vi "Continuous B sweep.vi"(7 "Rate (T/min)":dbl=0.028 min=0.0 max=0.2, 8 "error in (no error)":errorcluster, 9 "Simulate/Run":enum16{"simulate mode", "run mode"}(ring)=enum."run mode", 10 "Min (start)":dbl=7.0 min=-8.0 max=8.0, 11 "Max (end)":dbl=-7.0 min=-8.0 max=8.0) -> (0 "error out":errorcluster)   [LabVIEW 2016, in "SweepControl.lvclass"]
uses:
  SweepControl.lvclass
  Typedefs/Enum - Experiments.ctl
  Typedefs/Continuous B Sweep JSON--Cluster.ctl
  <userlib>/LevyLab/Levylab Instruments/Instrument Types/Cryostat/Instrument.Cryostat.lvclass
  Transport/Transport.lvclass
  Control Experiment/Control Experiment SM.lvclass
  <userlib>/LevyLab/Krohn Hite 7008/Instrument.KH7008.lvclass
  <userlib>/LevyLab/Lockin-Multichannel/Instrument.Lockin/Instrument.Lockin.lvclass
  Control Experiment/Typedefs/Instruments--cluster.ctl
  <userlib>/LevyLab/Krohn Hite 7008/typedefs/Input Configuration-Enum.ctl
  <userlib>/LevyLab/Krohn Hite 7008/typedefs/Shunt-Enum.ctl
  <userlib>/LevyLab/Krohn Hite 7008/typedefs/Gain-Enum.ctl
  <userlib>/LevyLab/Krohn Hite 7008/typedefs/Channel-Enum.ctl
  Control Experiment/Typedefs/Wiring Description--cluster.ctl
  Control Experiment/Typedefs/Instrument--enum.ctl
  Control Experiment/Typedefs/Experiment Description--cluster.ctl
  <userlib>/LevyLab/Levylab Instruments/Instrument Types/VSource/Instrument.VSource.lvclass
  <userlib>/LevyLab/Levylab Instruments/Instrument Types/VNA/Instrument.VNA.lvclass
  <userlib>/LevyLab/Levylab Instruments/Instrument Types/Strain/Instrument.Strain.lvclass
  <userlib>/LevyLab/Levylab Instruments/Instrument Types/Optical Delay Line/Instrument.OpticalDelayLine.lvclass
  <userlib>/LevyLab/Levylab Instruments/Instrument Types/CBridge/Instrument.CBridge.lvclass
  <userlib>/LevyLab/Krohn Hite 7008/typedefs/Coupling-Enum.ctl
  <userlib>/LevyLab/Krohn Hite 7008/typedefs/Filter-Enum.ctl
  <userlib>/LevyLab/Krohn Hite 7008/typedefs/SetAll-Cluster.ctl
  <userlib>/LevyLab/Krohn Hite 7008/typedefs/SetAll-Array.ctl
  <userlib>/LevyLab/Lockin-Multichannel/Lockin.DAQ/Typedefs/REF-cluster.ctl
  <userlib>/LevyLab/Lockin-Multichannel/Lockin.DAQ/Lockin.DAQ.lvclass
  <userlib>/LevyLab/Lockin-Multichannel/Lockin.DAQ/Typedefs/Function-enum.ctl
  <userlib>/LevyLab/Lockin-Multichannel/Lockin.DAQ/Typedefs/AO-cluster.ctl
  Typedefs/Lockin Sweep--Cluster.ctl
panel:
  in  "Sweep Lockin Array":T1[](array[typedef]) {"Sweep End (V)" format="%#_6p"; "Sweep Start (V)" format="%#_6p"}
  out "Current Setpoint":dbl
  in  "Experiment Folder":string="4L4Lockinfieldsweep"
  in  "Experiment subVI":T2
  in  "Experiment Description":string="SA03036H\nsweep Vsg:-150m to 700m, 500u steps\nB 7T to -7T\nVbg =-3.9V\nT: 50mK\n\nlockin\n\nI+/-: 4/28 200uV ac+ 250u dc bias, 13Hz\nV1+/-: 3/27\nV2+/- 2/6\nV3+/V3-: 7/8\nVsg: 1\nVbg :26\n\ntc 300ms order 2"
  in  "OK":bool
  out "time (minutes)":dbl
  out "ETA":timestamp=timestamp(3224621726.1089997 s since 1904-01-01) caption="Timestamp" format="%<%m/%d/%Y %I:%M:%S %p>T"
  out "time (hours)":dbl
  out "Current Step":i32
  in  "Function":enum16{"Ramp", "Triangle", "Sine"}(ring)
  in  "Phase":dbl
  in  "Cycles (1,2,...)":i32=1 min=1 step=1
  in  "step size":dbl=14.0 format="%.4f"
  out "B Field Graph":cluster{i32[], dbl[]}[](graph)
  in  "stop":bool
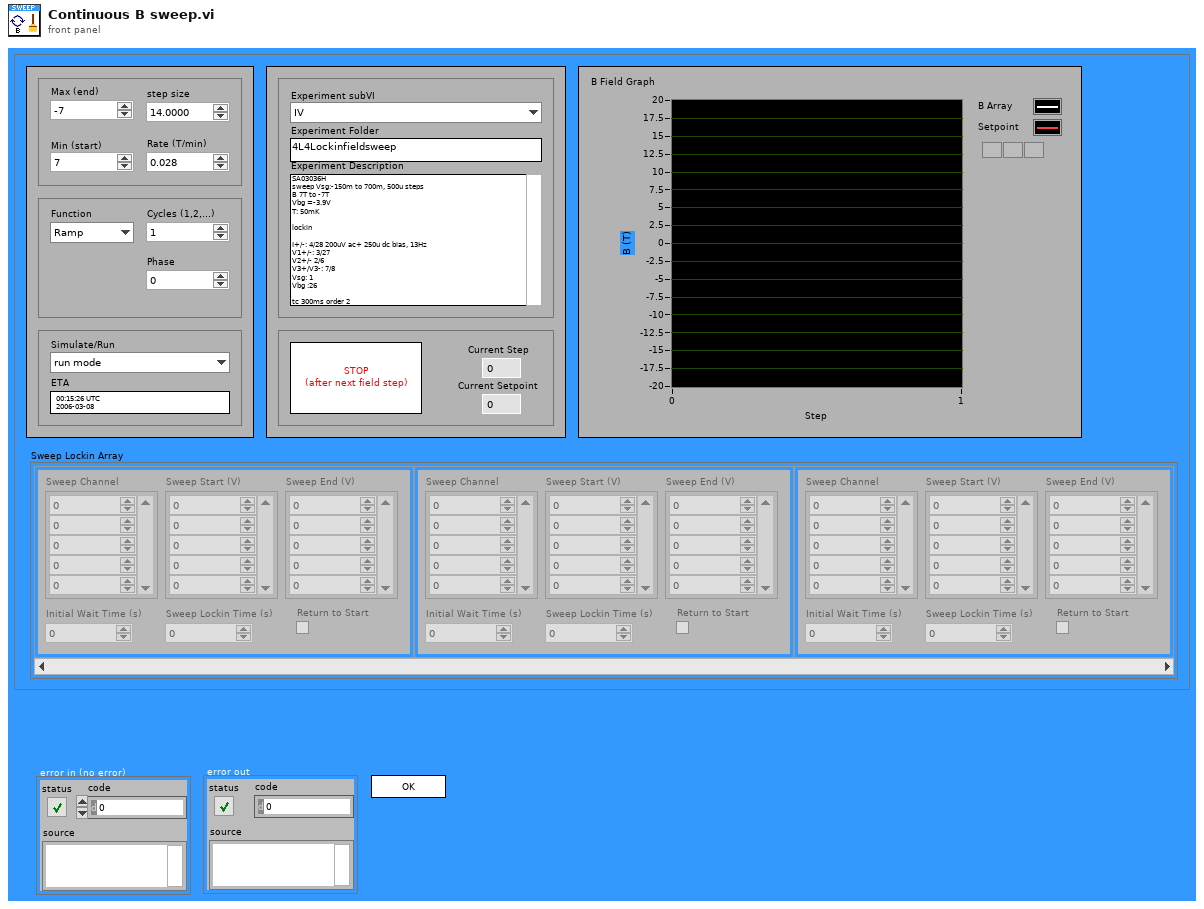
[diagram p1: front panel]
types:
  T1 = typedef "SweepControl.lvclass/Lockin Sweep--Cluster.ctl" = cluster{"Sweep Lockin Time (s)":dbl, "Initial Wait Time (s)":dbl, "Sweep Channel":i32[], "Sweep Start (V)":dbl[], "Sweep End (V)":dbl[], "Return to Start":bool}
  T2 = typedef "SweepControl.lvclass/Enum - Experiments.ctl" = enum16{"IV", "IV_Fast", "IV_Sweep", "THz_DelayLine", "Lockin_Vsg", "Lockin_Sweep", "Lockin_Time", "AI WFM time", "Lockin (experimental)"}
  T3 = enum32{"Invalid", "Standard", "Closed", "Hidden", "Minimized", "Maximized"}
  T4 = enum32{"invalid app kind", "Development System", "Run Time System", "Student Edition", "Embedded LabVIEW", "Evaluation", "Custom"}
  T5 = typedef "Control Experiment SM.lvclass/Instruments--cluster.ctl" = cluster{"KH7008":refnum<class "Instrument.KH7008.lvclass">[], "Lockin":refnum<class "Instrument.Lockin.lvclass">, "Temperature":refnum<class "Instrument.Cryostat.lvclass">, "Magnet":refnum<class "Instrument.Cryostat.lvclass">, "Rotator":refnum<class "Instrument.Cryostat.lvclass">, "Level":refnum<class "Instrument.Cryostat.lvclass">, "Capacitance Bridge":refnum<class "Instrument.CBridge.lvclass">, "Optical Delay Line":refnum<class "Instrument.OpticalDelayLine.lvclass">, "Strain Cell":refnum<class "Instrument.Strain.lvclass">, "VNA":refnum<class "Instrument.VNA.lvclass">, "Voltage Source":refnum<class "Instrument.VSource.lvclass">}
  T6 = cluster{"Core":cluster{"Current VI Reference":refnum<vi>, "Close Panel on Exit?":bool}, "SweepControl":refnum<class "SweepControl.lvclass">, "B field values":dbl[], "Sweep rate (T/min)":dbl, "Transport":refnum<class "Transport.lvclass">, "Instruments":T5, "Notifier":refnum<notifier>}
  T7 = cluster{"Current VI Reference":refnum<vi>, "Close Panel on Exit?":bool}
  T8 = typedef "SweepControl.lvclass/Continuous B Sweep JSON--Cluster.ctl" = cluster{"Continuous B Sweep":cluster{"Experiment":T2, "B field values":dbl[]}, "Experiment Description":T9, "Wiring Configuration":T11, "Lockin":cluster{"Channels: AO":T12, "Channels: Lockin":T14}, "Krohn Hite":cluster{"Channel Setting":T15}}
  T9 = typedef "Control Experiment SM.lvclass/Experiment Description--cluster.ctl" = cluster{"User":string, "Device":string, "Device Path":path, "Device Description":string, "Experiment Path":path, "Experiment Description":string, "Instrument":T10, "Sweep":cluster{"key":string, "value":variant}[], "Device Description JSON":string, "Experiment Description JSON":string}
  T10 = typedef "Control Experiment SM.lvclass/Instrument--enum.ctl" = enum16{"----- AFM/EBL -----", "AGILENT", "CYPHER", "Gemini2", "JEOL", "MFP3D", "----- Cryostat -----", "CF900", "DR200", "MNK", "PPMS 1", "PPMS 2", "PPMS 3", "----- Optics -----", "THz 1", "THz 2"}
  T11 = typedef "Control Experiment SM.lvclass/Wiring Description--cluster.ctl" = cluster{"Lockin Ch":i32[], "KH":cluster{"Electrodes":string[], "Labels":string[]}, "not KH":cluster{"Electrodes":string[], "Labels":string[]}}
  T12 = typedef "Lockin.DAQ.lvclass/AO-cluster.ctl" = cluster{"Ch":i32[], "Amp (V)":dbl[], "DC (V)":dbl[], "f (Hz)":dbl[], "Phase (°)":dbl[], "Function":T13[], "Sweep?":bool[]}
  T13 = typedef "Lockin.DAQ.lvclass/Function-enum.ctl" = enum16{"Sine", "Triangle", "Square", "Sawtooth"}
  T14 = typedef "Lockin.DAQ.lvclass/REF-cluster.ctl" = cluster{"Ch":i32[], " f (Hz)":dbl[], "Phase (°)":dbl[], "TC (s)":dbl[], "order":i32[]}
  T15 = typedef "Instrument.KH7008.lvclass/SetAll-Array.ctl" = T16[]
  T16 = typedef "Instrument.KH7008.lvclass/SetAll-Cluster.ctl" = cluster{"Channel":T17, "Gain":T18, "Bandwidth Filter":T19, "Shunt Resistor":T20, "Coupling":T21, "Input Config":T22}
  T17 = typedef "Instrument.KH7008.lvclass/Channel-Enum.ctl" = enum16{"Channel 1", "Channel 2", "Channel 3", "Channel 4", "Channel 5", "Channel 6", "Channel 7", "Channel 8"}
  T18 = typedef "Instrument.KH7008.lvclass/Gain-Enum.ctl" = enum16{"1x", "10x", "100x", "1000x"}
  T19 = typedef "Instrument.KH7008.lvclass/Filter-Enum.ctl" = enum16{"OFF", "ON"}
  T20 = typedef "Instrument.KH7008.lvclass/Shunt-Enum.ctl" = enum16{"Open", "50 Ohms", "500 Ohms", "5k Ohms", "50k Ohms", "10M Ohm"}
  T21 = typedef "Instrument.KH7008.lvclass/Coupling-Enum.ctl" = enum16{"AC", "DC"}
  T22 = typedef "Instrument.KH7008.lvclass/Input Configuration-Enum.ctl" = enum16{"Ground", "SE+ (-gnd)", "SE- (+gnd)", "Differential"}
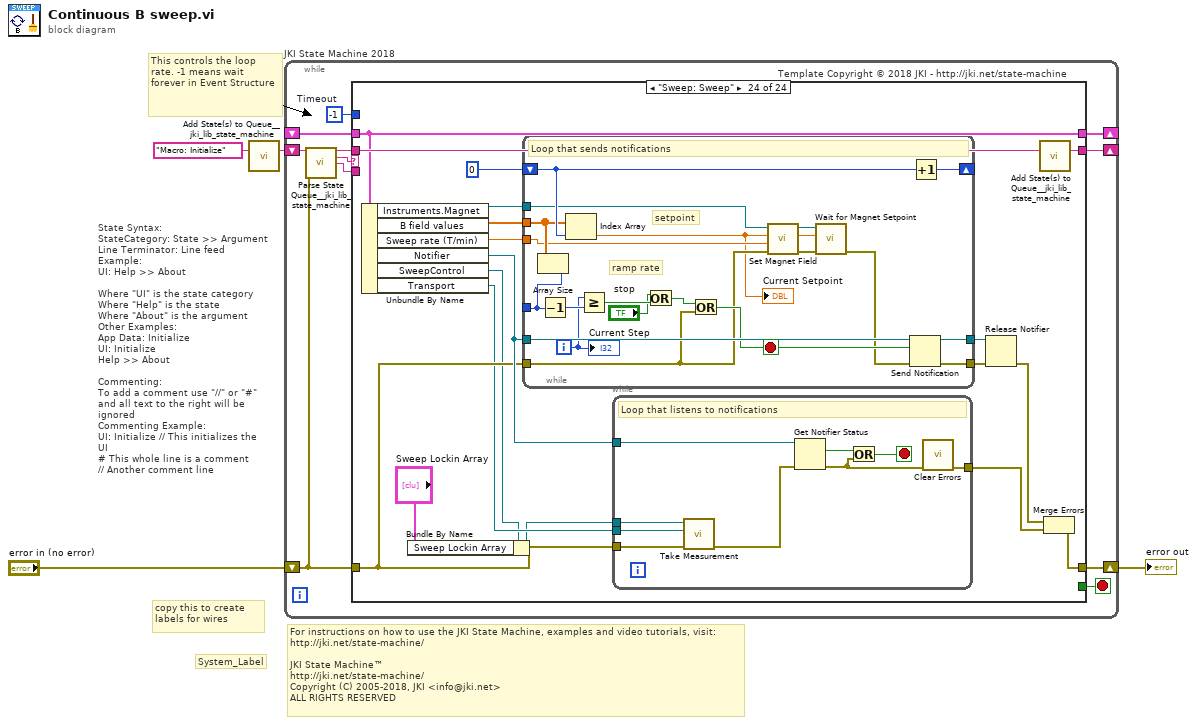
[diagram p0: block diagram]
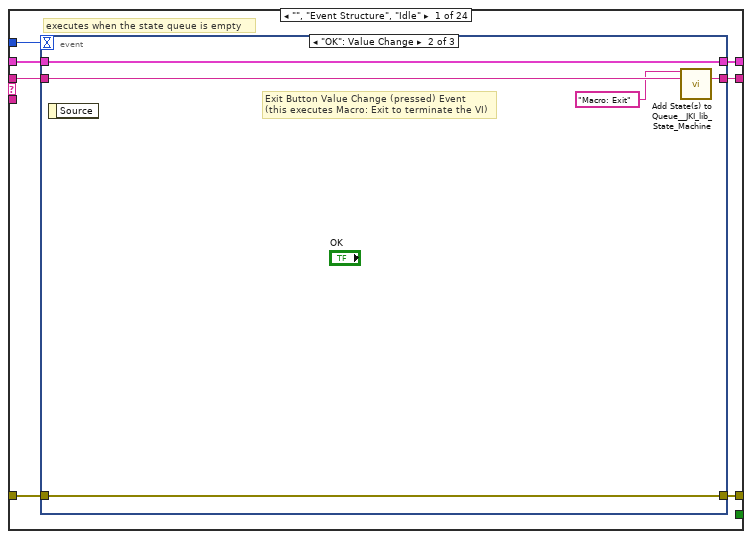
[diagram p2: hidden frame]
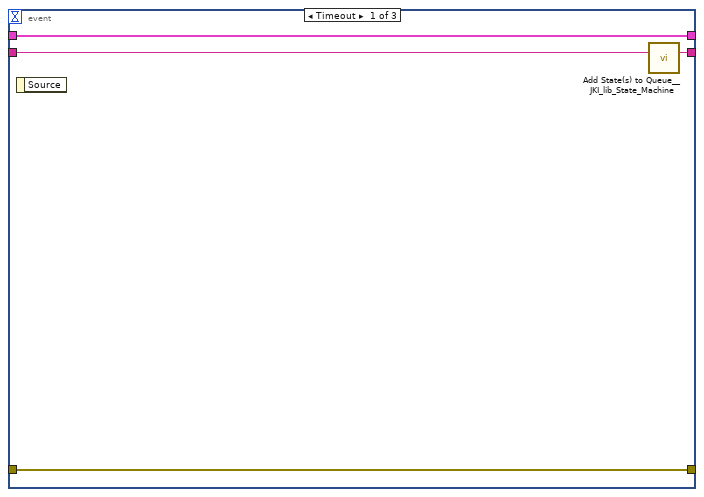
[diagram p3: hidden frame]
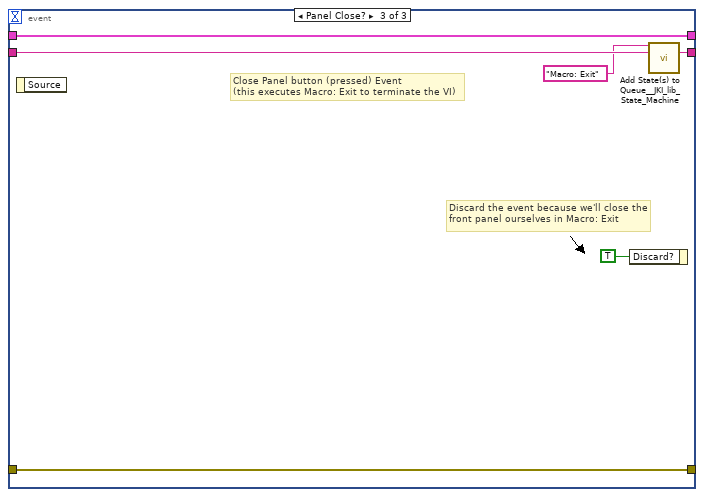
[diagram p4: hidden frame]
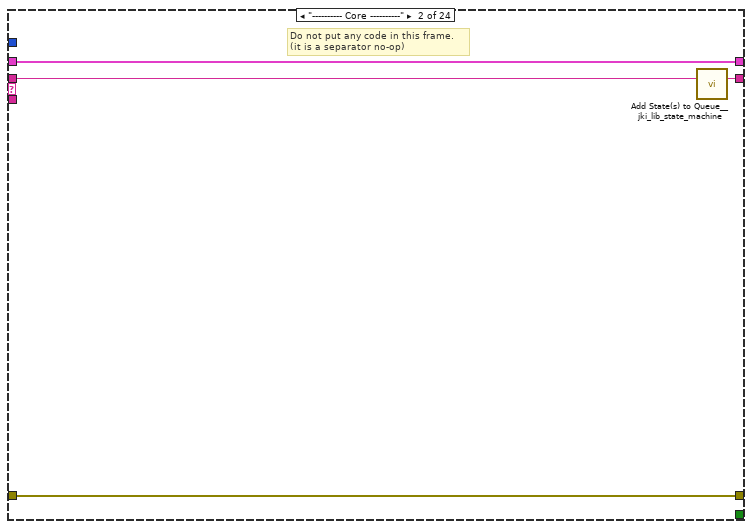
[diagram p5: hidden frame]
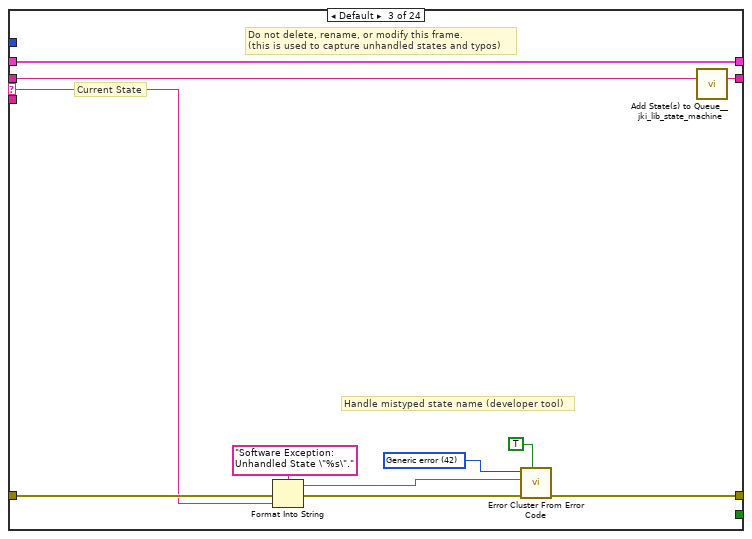
[diagram p6: hidden frame]
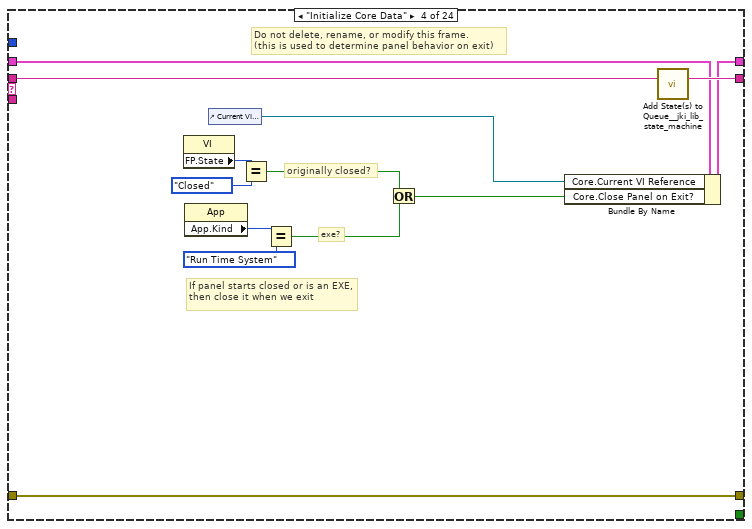
[diagram p7: hidden frame]
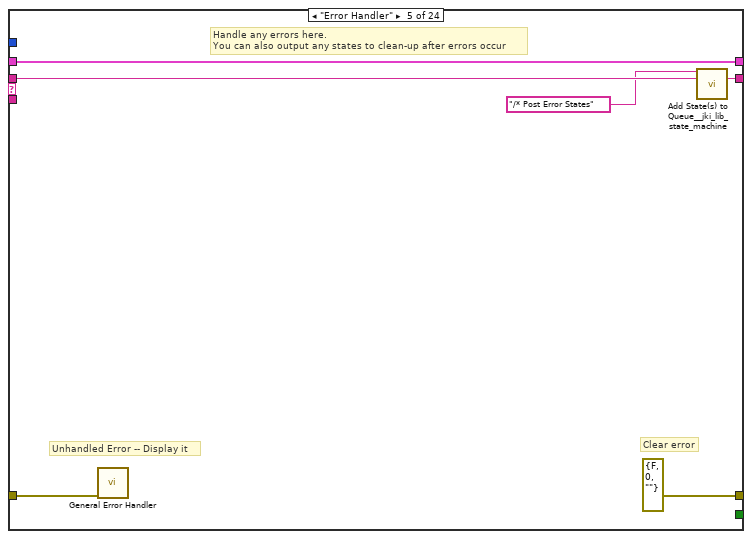
[diagram p8: hidden frame]
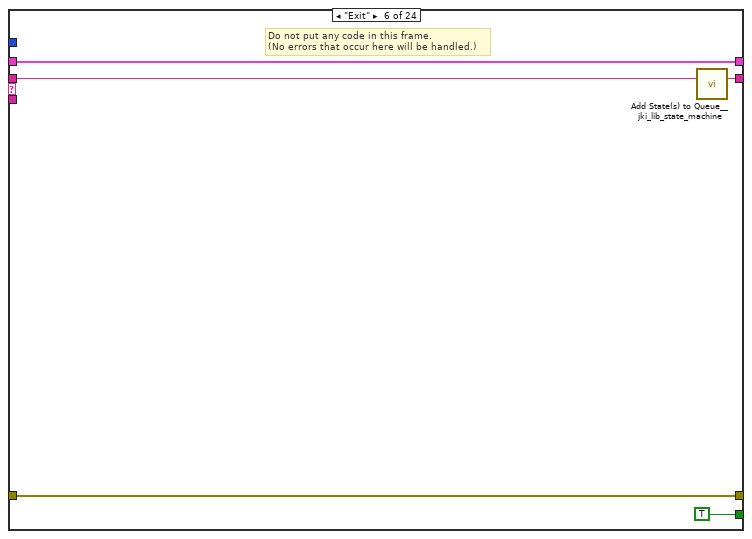
[diagram p9: hidden frame]
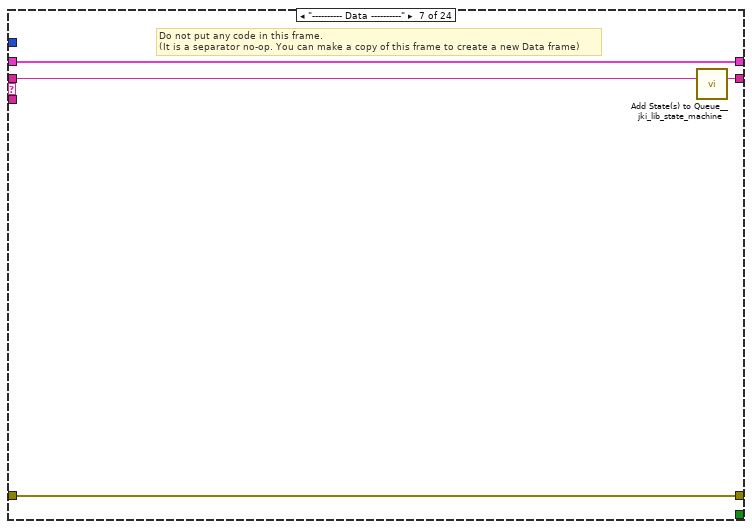
[diagram p10: hidden frame]
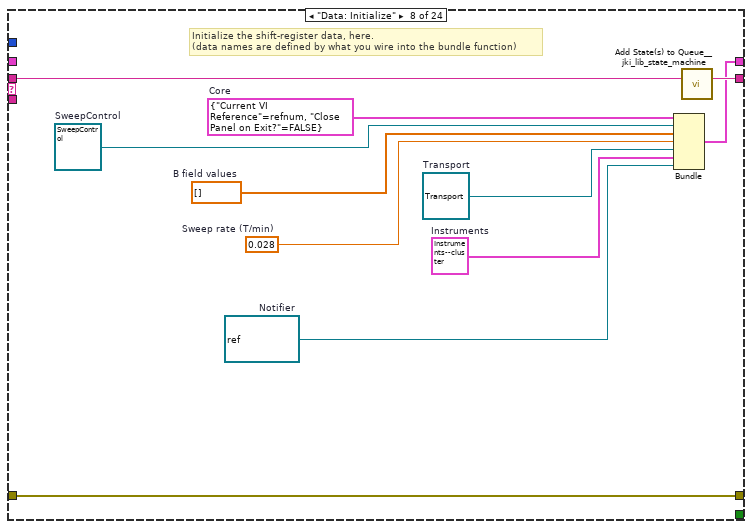
[diagram p11: hidden frame]
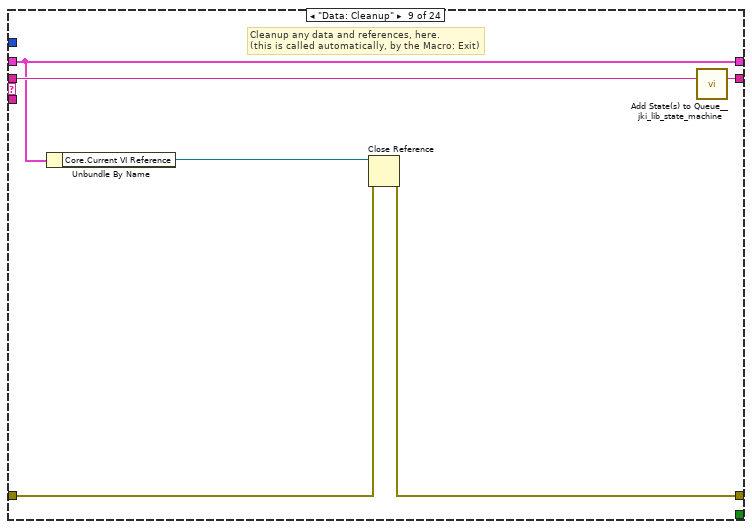
[diagram p12: hidden frame]
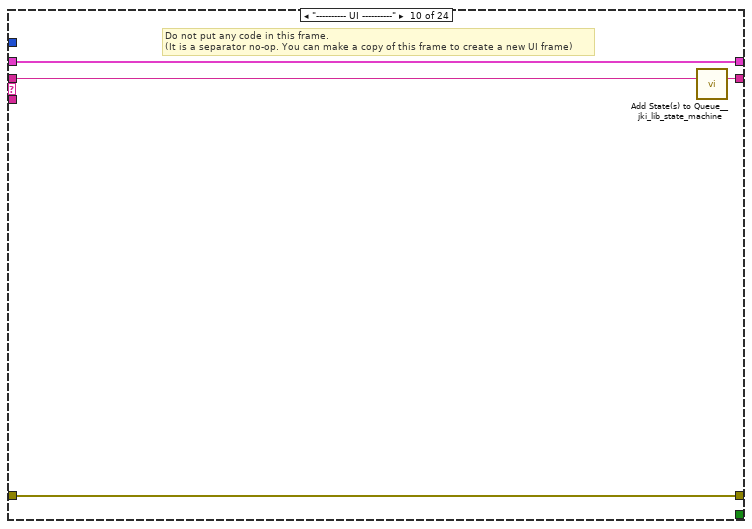
[diagram p13: hidden frame]
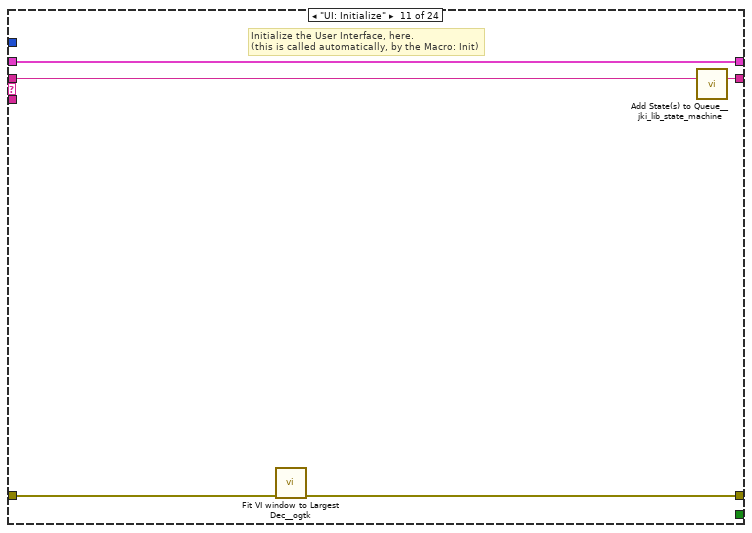
[diagram p14: hidden frame]
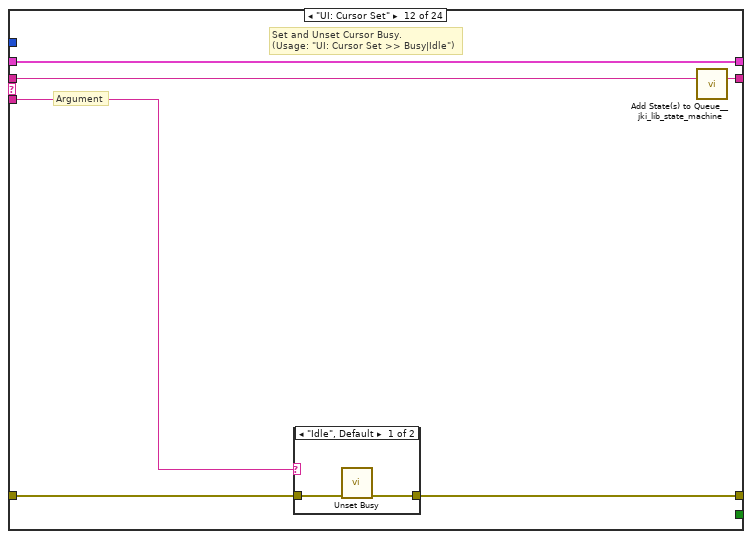
[diagram p15: hidden frame]
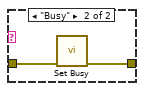
[diagram p16: hidden frame]
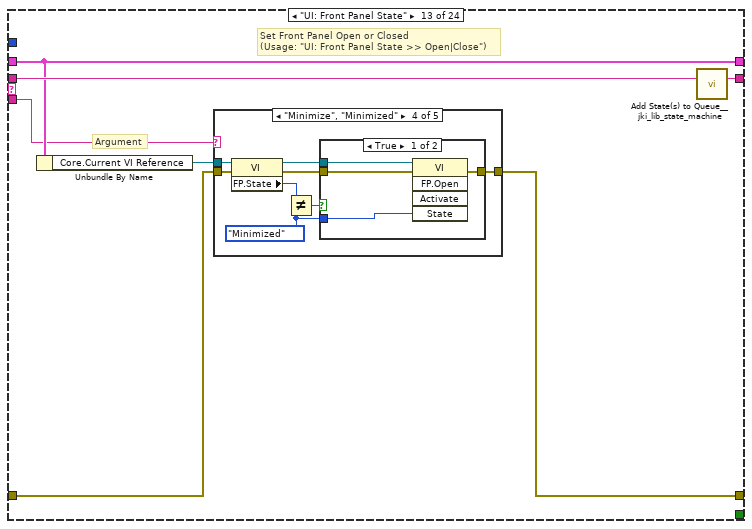
[diagram p17: hidden frame]
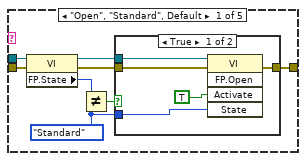
[diagram p18: hidden frame]
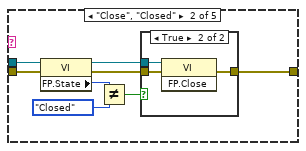
[diagram p20: hidden frame]
diagram:
  # "For instructions on how to use the JKI State Machine, examples and video tutorials, visit:\nhttp://jki.net/state-machine/\n\nJKI State Machine™\nhttp://jki.net/state-machine/\nCopyright (C) 2005-2018, JKI <info@jki.net>\nALL RIGHTS RESERVED"
  # "State Syntax:\nStateCategory: State >> Argument\nLine Terminator: Line feed\nExample:\nUI: Help >> About\n\nWhere \"UI\" is the state category\nWhere \"Help\" is the state\nWhere \"About\" is the argument\nOther Examples:\nApp Data: Initialize\nUI: Initialize\nHelp >> About\n\nCommenting:\nTo add a comment use \"//\" or \"#\" and all text to the right will be ignored\nCommenting Example:\nUI: Initialize // This initializes the UI\n# This whole line is a comment\n// Another comment line"
  # "copy this to create labels for wires"
  # "This controls the loop rate. -1 means wait forever in Event Structure"
  # "System_Label"
  n1 = call <vilib>:"Add State(s) to Queue__jki_lib_state_machine.vi"("State(s) in (\"\")"="Macro: Initialize") -> ("States Out"=w4:string)  [unwired: 14 in]
  n2 = while "JKI State Machine 2018" {
    shift-right: [w8] -> _
    shift-left: _ -> [w7]
    shift-right: [w11] -> w1
    shift-left: "error in (no error)" -> [w5]
    shift-right: [w10] -> _
    shift-left: w4 -> [w12]
    stop <- w9 stop-if-true
    w6 = -1  # Timeout
    # "Template Copyright © 2018 JKI - http://jki.net/state-machine"
    n3 = call <vilib>:"Parse State Queue__jki_lib_state_machine.vi"("State Queue"=w12, "Error In (no error)"=w5) -> ("Remaining States"=w14:string, "Current State"=w15:string, "Arguments"=w13:string)  [unwired: 11 in]
    n4 = case shown="\"Sweep: Sweep\"" w15 {
      selector: w15 -> [_ _ w42 _ _ _ _ _ _ _ _ _ _ _ _ _ _ _ _ _ _ _ _ _]
      tunnel: w14 -> [w22 w41 w46 w65 w71 w76 w80 w91 w97 w101 w106 w112 w123 w192 w197 w203 w215 w219 w238 w260 w274 w300 w321 w357]
      tunnel: w13 -> [_ _ _ _ _ _ _ _ _ _ _ w107 w117 _ _ _ _ _ _ _ _ _ _ _]
      tunnel: w7 -> [w20 w38 w44 w58 w68 w74 w77 _ w92 w98 w104 w110 w119 w189 w194 w200 w212 w216 w228 w244 w269 w298 w308 w349]
      tunnel: [w19 w39 w48 w62 errorcluster {"status"=FALSE, "code"=0, "source"=""} ("error out") w73 w78 w88 w93 w99 w102 w108 w120 w190 w195 w201 w213 w217 w226 w248 w267 w295 w319 w350] -> w11
      tunnel: w5 -> [w18 w39 w47 w62 w67 w73 w78 w88 w94 w99 w103 w109 w121 w190 w195 w201 w213 w217 w226 w249 w268 w282 w319 w344]
      tunnel: [w21 w40 w45 w64 w70 w75 w79 w90 w96 w100 w105 w111 w122 w191 w196 w202 w214 w218 w237 w259 w273 w299 w320 w356] -> w10
      tunnel: [_ _ _ _ _ TRUE _ _ _ _ _ _ _ _ _ _ _ _ _ _ _ _ _ _] -> w9
      tunnel: [w17 w38 w44 w63 w68 w74 w77 w89 w92 w98 w104 w110 w119 w189 w194 w200 w212 w216 w236 w243 w270 w298 w308 w349] -> w8
      tunnel: w6 -> [w16 _ _ _ _ _ _ _ _ _ _ _ _ _ _ _ _ _ _ _ _ _ _ _]
      frame "", "Event Structure", "Idle" {
        # "executes when the state queue is empty"
        n5 = event shown="[1] \"OK\": Value Change" {
          selector: _ -> [_ _ _]
          dyn-events: _ -> [_ _ _]
          timeout: w16 -> [_ _ _]
          tunnel: w22 -> [w26 w31 w37]
          tunnel: [w25 w30 w36] -> w21
          tunnel: w20 -> [w23 w28 w34]
          tunnel: [w24 w29 w35] -> w19
          tunnel: w18 -> [w24 w29 w35]
          tunnel: [w23 w28 w34] -> w17
          event Timeout {
            n6 = event-data() -> ()  [unwired: 1 in, 1 out]
            n7 = call <vilib>:"Add State(s) to Queue__JKI_lib_State_Machine.vi"("State(s) in (\"\")"=w26) -> ("States Out"=w25:string)  [unwired: 14 in]
          }
          event "OK": Value Change {
            # "Exit Button Value Change (pressed) Event\n(this executes Macro: Exit to terminate the VI)"
            n8 = event-data() -> ()  [unwired: 1 in, 1 out]
            n9 = call <vilib>:"Add State(s) to Queue__JKI_lib_State_Machine.vi"("State(s) in Front (\"\")"="Macro: Exit", "State(s) in (\"\")"=w31) -> ("States Out"=w30:string)  [unwired: 13 in]
          }
          event Panel Close? {
            # "Discard the event because we'll close the front panel ourselves in Macro: Exit"
            # "Close Panel button (pressed) Event\n(this executes Macro: Exit to terminate the VI)"
            n10 = event-data() -> ()  [unwired: 1 in, 1 out]
            n11 = event-data("Discard?"=TRUE) -> ()  [unwired: 1 in, 1 out]
            n12 = call <vilib>:"Add State(s) to Queue__JKI_lib_State_Machine.vi"("State(s) in Front (\"\")"="Macro: Exit", "State(s) in (\"\")"=w37) -> ("States Out"=w36:string)  [unwired: 13 in]
          }
        }
      }
      frame "---------- Core ----------" {
        # "Do not put any code in this frame.\n(it is a separator no-op)"
        n13 = call <vilib>:"Add State(s) to Queue__jki_lib_state_machine.vi"("State(s) in (\"\")"=w41) -> ("States Out"=w40:string)  [unwired: 14 in]
      }
      frame Default {
        w51 = 42 items=["No error", "Argument error", "Memory is full", "Out of zone", "End of file", "File already open", "Generic file I/O error", "File not found", "File permission error", "Disk is full", "Duplicate path", "Too many files open", "System feature not enabled", "Resource file not found", "Cannot add resource", "Resource not found", "Image not found", "Image memory error", "Pen does not exist", "Config type invalid", "Config token not found", "Config parse error", "Config memory error", "Bad external code format", "Bad external code offset", "External code not present", "Null window", "Destroy window error", "Null menu", "Print aborted", "Bad print record", "Print driver error", "Windows error during printing", "Memory error during printing", "Print dialog error", "Generic print error", "Invalid device refnum", "Device not found", "Device parameter error", "Device unit error", "Cannot open device", "Device call aborted", "Generic error", "Cancelled by user", "Object ID too low", "Object ID too high", "Object not in heap", "Unknown heap", "Unknown object (invalid DefProc)", "Unknown object (DefProc not in table)", "Message out of range", "Invalid (null) method", "Unknown message", "Manager call not supported", "Bad address", "Network operation in progress", "Network operation timed out", "Connection is busy", "Network attribute not supported", "Network error", "Address in use", "System out of memory", "Connection aborted", "Connection refused", "Not connected", "Already connected", "Connection closed", "Initialization error (interapplication manager)", "Bad occurrence", "Wait on unbound occurrence handler", "Occurrence queue overflow", "Datalog type conflict", "Unused", "Unrecognized type (interapplication manager)", "Memory corrupt", "Failed to make temporary DLL", "Old CIN version", "Drag socket not found", "Failed to load drop-object", "Failed to register OLE object", "Failed to release OLE object", "Format specifier type mismatch", "Unknown format specifier", "Too few format specifiers", "Too many format specifiers", "Scan failed", "Newer CIN version", "Error converting to variant", "Runtime menu error", "Password tampered", "Variant attribute not found", "Incompatible variant data type", "Event data is not available", "Event Store is not present", "Occurrence is not found", "Event Queue is not created", "Event info is not available", "Refnum passed is NULL", "Error retrieving Class GUID", "Error retrieving CoClass GUID", "Error retrieving TypeLib GUID.", "Bad built application magic bytes.", "Specific driver is different from the specific driver associated with the Logical Name.", "There is no session opened to the class driver.", "Max Error", "MAX - Error with config objects", "MAX - Error loading configuration", "MAX - Group not supported"]
        # "Current State"
        # "Do not delete, rename, or modify this frame.\n(this is used to capture unhandled states and typos)"
        # "Handle mistyped state name (developer tool)"
        n14 = Format Into String(format string="Software Exception: Unhandled State \"%s\"." ("message"), error in=w47, w42) -> (resulting string=w50:string, error out=w49:errorcluster)  [unwired: 1 in]
        n15 = call <vilib>:"Error Cluster From Error Code.vi"("show call chain? (False)"=TRUE, "error in (no error)"=w49, "error message (\"\")"=w50, "error code (0)"=w51) -> ("error out"=w48:errorcluster)  [unwired: 5 in]
        n16 = call <vilib>:"Add State(s) to Queue__jki_lib_state_machine.vi"("State(s) in (\"\")"=w46) -> ("States Out"=w45:string)  [unwired: 14 in]
      }
      frame "Initialize Core Data" {
        # "Do not delete, rename, or modify this frame.\n(this is used to determine panel behavior on exit)"
        # "originally closed?"
        # "exe?"
        # "If panel starts closed or is an EXE, then close it when we exit"
        n17 = property class="VI"() -> ("FP.State"=w55:T3)  [unwired: 2 in, 2 out]
        n18 = property class="App"() -> ("App.Kind"=w61:T4)  [unwired: 2 in, 2 out]
        n19 = control-ref of="Current VI Reference"() -> (w56:refnum<vi>)
        n20 = Equal?(x=w55, y=T3."Closed" ("Front Panel Window:State")) -> (x = y?=w53:bool)
        n21 = Equal?(x=w61, y=T4."Run Time System" ("Application:Kind")) -> (x = y?=w59:bool)
        n22 = Or(x=w53, y=w59) -> (x .or. y?=w57:bool)
        n23 = Bundle By Name(cluster=w58, "Core.Current VI Reference"=w56, "Core.Close Panel on Exit?"=w57) -> (w63:T6)
        n24 = call <vilib>:"Add State(s) to Queue__jki_lib_state_machine.vi"("State(s) in (\"\")"=w65) -> ("States Out"=w64:string)  [unwired: 14 in]
      }
      frame "Error Handler" {
        # "Unhandled Error -- Display it"
        # "Handle any errors here.\nYou can also output any states to clean-up after errors occur"
        # "Clear error"
        n25 = call <vilib>:"General Error Handler.vi"("error in (no error)"=w67) -> ()  [unwired: 10 in, 5 out]
        n26 = call <vilib>:"Add State(s) to Queue__jki_lib_state_machine.vi"("State(s) in Front (\"\")"="/* Post Error States", "State(s) in (\"\")"=w71) -> ("States Out"=w70:string)  [unwired: 13 in]
      }
      frame "Exit" {
        # "Do not put any code in this frame.\n(No errors that occur here will be handled.)"
        n27 = call <vilib>:"Add State(s) to Queue__jki_lib_state_machine.vi"("State(s) in (\"\")"=w76) -> ("States Out"=w75:string)  [unwired: 14 in]
      }
      frame "---------- Data ----------" {
        # "Do not put any code in this frame.\n(It is a separator no-op. You can make a copy of this frame to create a new Data frame)"
        n28 = call <vilib>:"Add State(s) to Queue__jki_lib_state_machine.vi"("State(s) in (\"\")"=w80) -> ("States Out"=w79:string)  [unwired: 14 in]
      }
      frame "Data: Initialize" {
        w81 = T5 {"KH7008"=[], "Lockin"=refnum, "Temperature"=refnum, "Magnet"=refnum, "Rotator"=refnum, "Level"=refnum, "Capacitance Bridge"=refnum, "Optical Delay Line"=refnum, "Strain Cell"=refnum, "VNA"=refnum, "Voltage Source"=refnum}  # Instruments
        w83 = refnum<class "Transport.lvclass"> refnum  # Transport
        w84 = refnum<class "SweepControl.lvclass"> refnum  # SweepControl
        w82 = refnum<notifier> refnum  # Notifier
        w85 = 0.028  # Sweep rate (T/min)
        w86 = dbl[] []  # B field values
        w87 = T7 {"Current VI Reference"=refnum, "Close Panel on Exit?"=FALSE}  # Core
        # "Initialize the shift-register data, here.\n(data names are defined by what you wire into the bundle function)"
        n29 = Bundle("Core"=w87, "SweepControl"=w84, "B field values"=w86, "Sweep rate (T/min)"=w85, "Transport"=w83, "Instruments"=w81, "Notifier"=w82) -> (w89:T6)  [unwired: 1 in]
        n30 = call <vilib>:"Add State(s) to Queue__jki_lib_state_machine.vi"("State(s) in (\"\")"=w91) -> ("States Out"=w90:string)  [unwired: 14 in]
      }
      frame "Data: Cleanup" {
        # "Cleanup any data and references, here.\n(this is called automatically, by the Macro: Exit)"
        n31 = Unbundle By Name(w92) -> ("Core.Current VI Reference"=w95:refnum<vi>)
        n32 = Close Reference(reference=w95, error in (no error)=w94) -> (error out=w93:errorcluster)
        n33 = call <vilib>:"Add State(s) to Queue__jki_lib_state_machine.vi"("State(s) in (\"\")"=w97) -> ("States Out"=w96:string)  [unwired: 14 in]
      }
      frame "---------- UI ----------" {
        # "Do not put any code in this frame.\n(It is a separator no-op. You can make a copy of this frame to create a new UI frame)"
        n34 = call <vilib>:"Add State(s) to Queue__jki_lib_state_machine.vi"("State(s) in (\"\")"=w101) -> ("States Out"=w100:string)  [unwired: 14 in]
      }
      frame "UI: Initialize" {
        # "Initialize the User Interface, here.\n(this is called automatically, by the Macro: Init)"
        n35 = call <userlib>:"Fit VI window to Largest Dec__ogtk.vi"("error in (no error)"=w103) -> ("error out"=w102:errorcluster)  [unwired: 5 in, 1 out]
        n36 = call <vilib>:"Add State(s) to Queue__jki_lib_state_machine.vi"("State(s) in (\"\")"=w106) -> ("States Out"=w105:string)  [unwired: 14 in]
      }
      frame "UI: Cursor Set" {
        # "Argument"
        # "Set and Unset Cursor Busy.\n(Usage: \"UI: Cursor Set >> Busy|Idle\")"
        n37 = case shown="\"Idle\", Default" w107 {
          tunnel: w109 -> [w114 w116]
          tunnel: [w113 w115] -> w108
          frame "Idle", Default {
            n38 = call <vilib>:"Unset Busy.vi"("error in (no error)"=w114) -> ("error out"=w113:errorcluster)  [unwired: 10 in]
          }
          frame "Busy" {
            n39 = call <vilib>:"Set Busy.vi"("error in (no error)"=w116) -> ("error out"=w115:errorcluster)  [unwired: 9 in, 1 out]
          }
        }
        n40 = call <vilib>:"Add State(s) to Queue__jki_lib_state_machine.vi"("State(s) in (\"\")"=w112) -> ("States Out"=w111:string)  [unwired: 14 in]
      }
      frame "UI: Front Panel State" {
        # "Argument"
        # "Set Front Panel Open or Closed\n(Usage: \"UI: Front Panel State >> Open|Close\")"
        n41 = Unbundle By Name(w119) -> ("Core.Current VI Reference"=w118:refnum<vi>)
        n42 = case shown="\"Minimize\", \"Minimized\"" w117 {
          tunnel: w121 -> [w129 w144 w155 w168 w181]
          tunnel: [w131 w145 w157 w170 w183] -> w120
          tunnel: w118 -> [w130 w142 w156 w169 w182]
          frame "Open", "Standard", Default {
            w124 = T3."Standard" ("State")
            n43 = property class="VI"(reference=w130, error in=w129) -> (reference out=w127:refnum<vi>, error out=w128:errorcluster, "FP.State"=w126:T3)
            n44 = Not Equal?(x=w126, y=w124) -> (x != y?=w125:bool)
            n45 = case shown="True" w125 {
              tunnel: [w135 w137] -> w131
              tunnel: w128 -> [w134 w137]
              tunnel: w127 -> [w133 _]
              tunnel: w124 -> [w132 _]
              frame True {
                n46 = invoke class="VI" method="FP.Open"(reference=w133, error in=w134, "Activate"=TRUE, "State"=w132) -> (error out=w135:errorcluster)  [unwired: 1 in, 4 out]
              }
              frame False {
              }
            }
          }
          frame "Close", "Closed" {
            n47 = property class="VI"(reference=w142, error in=w144) -> (reference out=w141:refnum<vi>, error out=w143:errorcluster, "FP.State"=w139:T3)
            n48 = Not Equal?(x=w139, y=T3."Closed" ("Front Panel Window:State")) -> (x != y?=w138:bool)
            n49 = case shown="True" w138 {
              tunnel: [w146 w149] -> w145
              tunnel: w143 -> [w146 w148]
              tunnel: w141 -> [_ w147]
              frame False {
              }
              frame True {
                n50 = invoke class="VI" method="FP.Close"(reference=w147, error in=w148) -> (error out=w149:errorcluster)  [unwired: 1 in, 2 out]
              }
            }
          }
          frame "Hidden", "Hide" {
            w150 = T3."Hidden" ("State")
            n51 = property class="VI"(reference=w156, error in=w155) -> (reference out=w153:refnum<vi>, error out=w154:errorcluster, "FP.State"=w152:T3)
            n52 = Not Equal?(x=w152, y=w150) -> (x != y?=w151:bool)
            n53 = case shown="True" w151 {
              tunnel: [w161 w162] -> w157
              tunnel: w154 -> [w160 w162]
              tunnel: w153 -> [w159 _]
              tunnel: w150 -> [w158 _]
              frame True {
                n54 = invoke class="VI" method="FP.Open"(reference=w159, error in=w160, "State"=w158) -> (error out=w161:errorcluster)  [unwired: 2 in, 4 out]
              }
              frame False {
              }
            }
          }
          frame "Minimize", "Minimized" {
            w163 = T3."Minimized" ("State")
            n55 = property class="VI"(reference=w169, error in=w168) -> (reference out=w166:refnum<vi>, error out=w167:errorcluster, "FP.State"=w165:T3)
            n56 = Not Equal?(x=w165, y=w163) -> (x != y?=w164:bool)
            n57 = case shown="True" w164 {
              tunnel: [w174 w175] -> w170
              tunnel: w167 -> [w173 w175]
              tunnel: w166 -> [w172 _]
              tunnel: w163 -> [w171 _]
              frame True {
                n58 = invoke class="VI" method="FP.Open"(reference=w172, error in=w173, "State"=w171) -> (error out=w174:errorcluster)  [unwired: 2 in, 4 out]
              }
              frame False {
              }
            }
          }
          frame "Maximize", "Maximized" {
            w176 = T3."Maximized" ("State")
            n59 = property class="VI"(reference=w182, error in=w181) -> (reference out=w179:refnum<vi>, error out=w180:errorcluster, "FP.State"=w178:T3)
            n60 = Not Equal?(x=w178, y=w176) -> (x != y?=w177:bool)
            n61 = case shown="True" w177 {
              tunnel: [w187 w188] -> w183
              tunnel: w180 -> [w186 w188]
              tunnel: w179 -> [w185 _]
              tunnel: w176 -> [w184 _]
              frame True {
                n62 = invoke class="VI" method="FP.Open"(reference=w185, error in=w186, "State"=w184) -> (error out=w187:errorcluster)  [unwired: 2 in, 4 out]
              }
              frame False {
              }
            }
          }
        }
        n63 = call <vilib>:"Add State(s) to Queue__jki_lib_state_machine.vi"("State(s) in (\"\")"=w123) -> ("States Out"=w122:string)  [unwired: 14 in]
      }
      frame "---------- Macro ----------" {
        # "Do not put any code in this frame.\n(It is a separator no-op. You can make a copy of this frame to create a new Macro frame)"
        n64 = call <vilib>:"Add State(s) to Queue__jki_lib_state_machine.vi"("State(s) in (\"\")"=w192) -> ("States Out"=w191:string)  [unwired: 14 in]
      }
      frame "Macro: Initialize" {
        w193 = "Data: Initialize\nInitialize Core Data\nUI: Initialize\nUI: Front Panel State >> Open\nMacro: Sweep"  # Data: Initialize Initialize Core Data UI: Initialize UI: Front Panel State >> Open Macro: Sweep
        # "Initialization Macro\n(This is called once, when the VI starts)"
        n65 = call <vilib>:"Add State(s) to Queue__jki_lib_state_machine.vi"("State(s) in Front (\"\")"=w193, "State(s) in (\"\")"=w197) -> ("States Out"=w196:string)  [unwired: 13 in]
      }
      frame "Macro: Sweep" {
        # "Do not put any code in this frame.\n(It is a separator no-op. You can make a copy of this frame to create a new Macro frame)"
        n66 = case shown="\"run mode\"" "Simulate/Run" {
          tunnel: ["Sweep: Initialize\nSweep: Simulate Sweep\nMacro: Exit" "Sweep: Initialize\nSweep: Initialize Sweep Control\nSweep: Initialize Transport\nSweep: Save JSON File\nSweep: Sweep\nMacro: Exit"] -> w199
          frame "simulate mode", Default {
          }
          frame "run mode" {
          }
        }
        n67 = call <vilib>:"Add State(s) to Queue__jki_lib_state_machine.vi"("State(s) in Front (\"\")"=w199, "State(s) in (\"\")"=w203) -> ("States Out"=w202:string)  [unwired: 13 in]
      }
      frame "Macro: Exit" {
        # "Exit Macro\n(This is called once, when the VI exits)"
        n68 = Unbundle By Name(w212) -> ("Core.Close Panel on Exit?"=w211:bool)
        n69 = Select(t="UI: Front Panel State >> Close", s=w211, f="") -> (s? t:f=w208:string)
        n70 = call <vilib>:"Add State(s) to Queue__JKI_lib_State_Machine.vi"("State(s) in (\"\")"=w208, "State(s) at Back (\"\")"="Data: Cleanup\nExit") -> ("States Out"=w206:string)  [unwired: 13 in]
        n71 = call <vilib>:"Add State(s) to Queue__jki_lib_state_machine.vi"("State(s) in Front (\"\")"=w206, "State(s) in (\"\")"=w215) -> ("States Out"=w214:string)  [unwired: 13 in]
      }
      frame "---------- Sweep ----------" {
        # "Template Separator\n(You can make a copy of, or modify, this frame)"
        n72 = call <vilib>:"Add State(s) to Queue__jki_lib_state_machine.vi"("State(s) in (\"\")"=w219) -> ("States Out"=w218:string)  [unwired: 14 in]
      }
      frame "Sweep: Initialize" {
        # "Your code here.\n(You can make a copy of, or modify, this frame)"
        n73 = call <userlib>:"Max_Min_conversion.vi"("Min"="Min (start)", "Max"="Max (end)") -> ("offset"=w231:dbl, "Amplitude"=w230:dbl)  [unwired: 8 in]
        n74 = call <userlib>:"Ramp.vi"("phase"="Phase", "function (ramp)"="Function", "cycles (1,2,...)"="Cycles (1,2,...)", "step size"="step size", "offset"=w231, "amplitude"=w230) -> ("Waveform Graph"=w224:dbl[])  [unwired: 3 in, 2 out]
        n75 = for {
          tunnel: w224 -> [w239] mode=indexing
          tunnel: [w240] -> w223 mode=indexing
          tunnel: [w239] -> w222 mode=indexing
          i -> [w240]
        }
        n76 = Bundle(w223, w222) -> (w221:cluster{i32[], dbl[]})  [unwired: 1 in]
        n77 = Build Array(w221) -> (→"B Field Graph":cluster{i32[], dbl[]}[])
        n78 = Bundle By Name(cluster=w228, "B field values"=w224, "Sweep rate (T/min)"="Rate (T/min)") -> (w236:T6)
        n79 = call <vilib>:"Add State(s) to Queue__jki_lib_state_machine.vi"("State(s) in (\"\")"=w238) -> ("States Out"=w237:string)  [unwired: 14 in]
      }
      frame "Sweep: Initialize Sweep Control" {
        # "Template Separator\n(You can make a copy of, or modify, this frame)"
        n80 = Unbundle By Name(w244) -> ("SweepControl"=w251:refnum<class "SweepControl.lvclass">)
        n81 = call "Control Experiment FGV.vi"("Function"=enum16{"read", "write"}."read", "error in (no error)"=w249) -> ("error out"=w245:errorcluster, "Control Experiment.lvclass out"=w256:refnum<class "Control Experiment SM.lvclass">)  [unwired: 8 in]
        n82 = call "Write Experiment Description.vi"("error in (no error)"=w245, "Experiment Description"="Experiment Description", "Control Experiment in"=w256) -> ("error out"=w246:errorcluster, "Control Experiment out"=w255:refnum<class "Control Experiment SM.lvclass">)  [unwired: 7 in]
        n83 = call "Write Experiment Folder.vi"("error in (no error)"=w246, "Experiment Folder"="Experiment Folder", "Control Experiment in"=w255) -> ("error out"=w247:errorcluster, "Control Experiment out"=w257:refnum<class "Control Experiment SM.lvclass">)  [unwired: 7 in]
        n84 = call "Read Instruments.vi"("error in (no error)"=w247, "Control Experiment in"=w257) -> ("error out"=w248:errorcluster, "Instruments"=w241:T5, "Control Experiment out"=w250:refnum<class "Control Experiment SM.lvclass">)  [unwired: 7 in]
        n85 = Bundle By Name(cluster=w251, "Experiment"="Experiment subVI", "Control Experiment"=w250) -> (w242:refnum<class "SweepControl.lvclass">)
        n86 = Bundle By Name(cluster=w244, "SweepControl"=w242, "Instruments"=w241) -> (w243:T6)
        n87 = call <vilib>:"Add State(s) to Queue__jki_lib_state_machine.vi"("State(s) in (\"\")"=w260) -> ("States Out"=w259:string)  [unwired: 14 in]
      }
      frame "Sweep: Initialize Transport" {
        # "Template Separator\n(You can make a copy of, or modify, this frame)"
        n88 = Unbundle By Name(w269) -> ("SweepControl"=w263:refnum<class "SweepControl.lvclass">)
        n89 = Obtain Notifier(notification data type=FALSE, error in (no error)=w268) -> (notifier out=w261:refnum<notifier>, error out=w265:errorcluster)  [unwired: 2 in, 1 out]
        n90 = call "Write Dependencies.vi"("error in (no error)"=w265, "SweepControl"=w263, "Transport in"=refnum<class "Transport.lvclass"> refnum) -> ("error out"=w266:errorcluster, "Transport out"=w271:refnum<class "Transport.lvclass">)  [unwired: 7 in]
        n91 = call "Write notifier.vi"("error in (no error)"=w266, "notifier"=w261, "Transport in"=w271) -> ("error out"=w267:errorcluster, "Transport out"=w264:refnum<class "Transport.lvclass">)  [unwired: 7 in]
        n92 = Bundle By Name(cluster=w269, "Transport"=w264, "Notifier"=w261) -> (w270:T6)
        n93 = call <vilib>:"Add State(s) to Queue__jki_lib_state_machine.vi"("State(s) in (\"\")"=w274) -> ("States Out"=w273:string)  [unwired: 14 in]
      }
      frame "Sweep: Save JSON File" {
        w297 = T8 {"Continuous B Sweep"={"Experiment"=enum."IV", "B field values"=[]}, "Experiment Description"={"User"="", "Device"="", "Device Path"=path "", "Device Description"="", "Experiment Path"=path "", "Experiment Description"="", "Instrument"=enum."PPMS 1", "Sweep"=[], "Device Description JSON"="", "Experiment Description JSON"=""}, "Wiring Configuration"={"Lockin Ch"=[], "KH"={"Electrodes"=[], "Labels"=[]}, "not KH"={"Electrodes"=[], "Labels"=[]}}, "Lockin"={"Channels: AO"={"Ch"=[], "Amp (V)"=[], "DC (V)"=[], "f (Hz)"=[], "Phase (°)"=[], "Function"=[], "Sweep?"=[]}, "Channels: Lockin"={"Ch"=[], " f (Hz)"=[], "Phase (°)"=[], "TC (s)"=[], "order"=[]}}, "Krohn Hite"={"Channel Setting"=[]}}  # ContinuousBSweep
        n94 = Unbundle By Name(w298) -> ("SweepControl"=w284:refnum<class "SweepControl.lvclass">, "B field values"=w285:dbl[], "Instruments.Lockin"=w292:refnum<class "Instrument.Lockin.lvclass">, "Instruments.KH7008"=w287:refnum<class "Instrument.KH7008.lvclass">[])
        n95 = Unbundle By Name(w284) -> ("Control Experiment"=w275:refnum<class "Control Experiment SM.lvclass">, "Experiment"=w276:T2)
        n96 = for {
          tunnel: w287 -> [w304] mode=indexing
          tunnel: [w302] -> w283 mode=concatenating
          tunnel: w282 -> [w301]
          tunnel: [w303] -> w277
          n97 = call <userlib>:"Read Channel Setting.vi"("error in (no error)"=w301, "Instrument.KH7008 in"=w304) -> ("error out"=w303:errorcluster, "Channel Setting"=w302:T15)  [unwired: 7 in, 1 out]
        }
        n98 = call "Read Experiment Configuration.vi"("error in (no error)"=w282, "Control Experiment in"=w275) -> ("error out"=w288:errorcluster, "Experiment Description"=w290:T9, "Control Experiment out"=w286:refnum<class "Control Experiment SM.lvclass">)  [unwired: 7 in]
        n99 = call <userlib>:"getAOconfig.vi"("error in (no error)"=w282, "Instrument.Lockin in"=w292) -> ("error out"=w293:errorcluster, "AOconfig"=w281:T12, "Instrument.Lockin out"=w294:refnum<class "Instrument.Lockin.lvclass">)  [unwired: 7 in]
        n100 = call "Read Wiring Configuration.vi"("error in (no error)"=w288, "Control Experiment in"=w286) -> ("error out"=w279:errorcluster, "Wiring Configuration"=w289:T11)  [unwired: 7 in, 1 out]
        n101 = call <userlib>:"getREFconfig.vi"("error in (no error)"=w293, "Instrument.Lockin in"=w294) -> ("error out"=w280:errorcluster, "REFconfig"=w291:T14)  [unwired: 7 in, 1 out]
        n102 = Bundle By Name(cluster=w297, "Continuous B Sweep.Experiment"=w276, "Continuous B Sweep.B field values"=w285, "Experiment Description"=w290, "Wiring Configuration"=w289, "Lockin.Channels: AO"=w281, "Lockin.Channels: Lockin"=w291, "Krohn Hite.Channel Setting"=w283) -> (w296:T8)
        n103 = Merge Errors(w279, w280, w277) -> (w278:errorcluster)
        n104 = call "Save JSON File.vi"("error in (no error)"=w278, "Data"=w296, "Control Experiment in"=w275) -> ("error out"=w295:errorcluster)  [unwired: 6 in, 2 out]
        n105 = call <vilib>:"Add State(s) to Queue__jki_lib_state_machine.vi"("State(s) in (\"\")"=w300) -> ("States Out"=w299:string)  [unwired: 14 in]
      }
      frame "Sweep: Simulate Sweep" {
        # "Sweep Rate"
        # "B Field Values"
        # "Template Separator\n(You can make a copy of, or modify, this frame)"
        n106 = Unbundle By Name(w308) -> ("Sweep rate (T/min)"=w307:dbl, "B field values"=w306:dbl[])
        n107 = Array Size(array=w306) -> (size(s)=w309:i32)
        n108 = Decrement(x=w309) -> (x-1=w310:i32)
        n109 = for {
          N: w310 -> [_]
          tunnel: w307 -> [w331]
          tunnel: w306 -> [w339]
          tunnel: [w332] -> w311 mode=indexing
          i -> [w337]
          n110 = Increment(x=w337) -> (x+1=w338:i32)
          n111 = Index Array(array=w339, index #1=w337, index #2=w338) -> (element #1=w335:dbl, element #2=w336:dbl)
          n112 = Subtract(x=w335, y=w336) -> (x-y=w334:dbl)
          n113 = Absolute Value(x=w334) -> (abs(x)=w333:dbl)
          n114 = Divide(x=w333, y=w331) -> (x/y=w332:dbl)
        }
        n115 = for {
          tunnel: w306 -> [w323] mode=indexing
          i -> [w324]
          n116 = local read "B Field Graph"() -> (w327:cluster{i32[], dbl[]}[])
          n117 = Build Array(w324) -> (w329:i32[])
          n118 = Build Array(w323) -> (w328:dbl[])
          n119 = Bundle(w329, w328) -> (w325:cluster{i32[], dbl[]})  [unwired: 1 in]
          n120 = local write "Current Setpoint"(w323) -> ()
          n121 = local write "Current Step"(w324) -> ()
          n122 = Index Array(array=w327) -> (element=w326:cluster{i32[], dbl[]})  [unwired: 1 in]
          n123 = Build Array(w326, w325) -> (w322:cluster{i32[], dbl[]}[])
          n124 = local write "B Field Graph"(w322) -> ()
          n125 = call <userlib>:"Wait (ms)__ogtk.vi"("milliseconds to wait"=u32 250) -> ()  [unwired: 9 in, 2 out]
        }
        n126 = Get Date/Time In Seconds() -> (seconds since 1Jan1904=w314:timestamp)
        n127 = Add Array Elements(numeric array=w311) -> (sum=w316:dbl)
        n128 = Quotient & Remainder(x=w316, y=60.0) -> (x-y*floor(x/y)=→"time (minutes)":dbl, floor(x/y)=→"time (hours)":dbl)
        n129 = Multiply(x=w316, y=60.0) -> (x*y=w313:dbl)
        n130 = Add(x=w313, y=w314) -> (x+y=→"ETA":timestamp)
        n131 = call <vilib>:"Add State(s) to Queue__jki_lib_state_machine.vi"("State(s) in (\"\")"=w321) -> ("States Out"=w320:string)  [unwired: 14 in]
      }
      frame "Sweep: Sweep" {
        n132 = Unbundle By Name(w349) -> ("Instruments.Magnet"=w345:refnum<class "Instrument.Cryostat.lvclass">, "B field values"=w346:dbl[], "Sweep rate (T/min)"=w347:dbl, "Notifier"=w348:refnum<notifier>, "SweepControl"=w342:refnum<class "SweepControl.lvclass">, "Transport"=w343:refnum<class "Transport.lvclass">)
        n133 = Bundle By Name(cluster=w342, "Sweep Lockin Array"="Sweep Lockin Array") -> (w341:refnum<class "SweepControl.lvclass">)
        n134 = while {
          tunnel: w348 -> [w384]
          tunnel: w344 -> [w371]
          tunnel: [w386] -> w355
          tunnel: [w385] -> w353
          shift-right: [w382] -> _
          shift-left: 0 -> [w379]
          tunnel: w346 -> [w376]
          tunnel: [w377] -> _
          tunnel: w347 -> [w375]
          tunnel: w345 -> [w369]
          i -> [w378]
          stop <- w374 stop-if-true
          # "setpoint"
          # "ramp rate"
          # "Loop that sends notifications"
          n135 = Array Size(array=w376) -> (size(s)=w377:i32)
          n136 = Decrement(x=w377) -> (x-1=w380:i32)
          n137 = Index Array(array=w376, index=w379) -> (element=w368:dbl)
          "Current Setpoint" <- w368
          n138 = Greater Or Equal?(x=w378, y=w380) -> (x >= y?=w381:bool)
          n139 = Or(x="stop", y=w381) -> (x .or. y?=w383:bool)
          n140 = Or(x=w383, y=w371) -> (x .or. y?=w374:bool)
          n141 = call-dynamic "Set Magnet Field.vi"("error in (no error)"=w371, "Target Rate (T/min)"=w375, "Target Field (T)"=w368, "Instrument.Cryostat in"=w369) -> ("error out"=w372:errorcluster, "Instrument.Cryostat out"=w373:refnum<class "Instrument.Cryostat.lvclass">)  [unwired: 6 in]
          n142 = call <userlib>:"Wait for Magnet Setpoint.vi"("error in (no error)"=w372, "Setpoint (T)"=w368, "Instrument.Cryostat in"=w373) -> ("error out"=w370:errorcluster)  [unwired: 7 in, 1 out]
          n143 = Send Notification(notification=w374, notifier=w384, error in (no error)=w370) -> (notifier out=w386:refnum<notifier>, error out=w385:errorcluster)
          n144 = Increment(x=w379) -> (x+1=w382:i32)
          "Current Step" <- w378
        }
        n145 = while {
          tunnel: w344 -> [w361]
          tunnel: w348 -> [w362]
          tunnel: [w363] -> w352
          tunnel: w341 -> [w359]
          tunnel: w343 -> [w358]
          stop <- w366 stop-if-true
          # "Loop that listens to notifications"
          n146 = call "Take Measurement.vi"("error in (no error)"=w361, "Transport in"=w358, "SweepControl in"=w359) -> ("error out"=w360:errorcluster)  [unwired: 5 in, 3 out]
          n147 = Get Notifier Status(notifier=w362, error in (no error)=w360) -> (current notification=w365:bool, error out=w364:errorcluster)  [unwired: 3 out]
          n148 = Or(x=w365, y=w364) -> (x .or. y?=w366:bool)
          n149 = call <vilib>:"Clear Errors.vi"("error in (no error)"=w364) -> ("error out"=w363:errorcluster)  [unwired: 5 in, 1 out]
        }
        n150 = Release Notifier(notifier=w355, error in (no error)=w353) -> (error out=w351:errorcluster)  [unwired: 1 in, 2 out]
        n151 = call <vilib>:"Add State(s) to Queue__jki_lib_state_machine.vi"("State(s) in (\"\")"=w357) -> ("States Out"=w356:string)  [unwired: 14 in]
        n152 = Merge Errors(w351, w352) -> (w350:errorcluster)
      }
    }
  }
  "error out" <- w1
